vi "LIN_Config.vi"(10 "Data":T2={"Communication message"={"Sender"="", "receiver"="", "message"="", "data"=variant}, "LIN_Data"={"DLL_PATH"=path "", "Channels used"=1, "Funtiontype"=0, "Rx/TX"=enum."Rx", "Read message type"=enum."Receive&send messages", "async&sync"=enum."async", "sync_sendTimeout"=0, "LIN_SendHead"={"ALINIdxchn"=0, "ALINId"=0, "ALINDLC"=0}, "LIN_Set"={"Hardware Type"=2, "Hardware Subtype"=enum."TC1016", "AHwChannel"=0, "AAppChannel"=19, "ABaudrateKbps"=19.2, "AProtocol"=2, "AldHW"=0}, "LIN_DATA"={"Data0"=0, "Data1"=0, "Data2"=0, "Data3"=0, "Data4"=0, "Data5"=0, "Data6"=0, "Data7"=0}, "LIN_Set_Array"=[], "LDF"={"LDF Path"=path "", "LDF loading channel"=0}, "Blf_Log"={"Blf_Log_PATH"=path ""}, "LIN Scheduling Table Array"=[], "REC_Channel"=0}, "LIN Data array"=[], "error in"={"status"=FALSE, "code"=0, "source"=""}, "REC_Channel"=0, "AsynCall?"=FALSE, "DataBase_array"=refnum} {"REC_Channel" items=["CHN1", "CHN2", "CHN3", "CHN4", "CHN5", "CHN6", "CHN7", "CHN8", "CHN9", "CHN10", "CHN11", "CHN12", "CHN13", "CHN14", "CHN15", "CHN16", "CHN17", "CHN18", "CHN19", "CHN20", "CHN21", "CHN22", "CHN23", "CHN24", "CHN25", "CHN26", "CHN27", "CHN28", "CHN29", "CHN30", "CHN31", "CHN32"]; "LIN_Data"."REC_Channel" items=["CHN1", "CHN2", "CHN3", "CHN4", "CHN5", "CHN6", "CHN7", "CHN8", "CHN9", "CHN10", "CHN11", "CHN12", "CHN13", "CHN14", "CHN15", "CHN16", "CHN17", "CHN18", "CHN19", "CHN20", "CHN21", "CHN22", "CHN23", "CHN24", "CHN25", "CHN26", "CHN27", "CHN28", "CHN29", "CHN30", "CHN31", "CHN32"]; "LIN_Data"."LIN Scheduling Table Array"."LIN_Transmit"."Channel" items=["CHN1", "CHN2", "CHN3", "CHN4", "CHN5", "CHN6", "CHN7", "CHN8", "CHN9", "CHN10", "CHN11", "CHN12", "CHN13", "CHN14", "CHN15", "CHN16", "CHN17", "CHN18", "CHN19", "CHN20", "CHN21", "CHN22", "CHN23", "CHN24", "CHN25", "CHN26", "CHN27", "CHN28", "CHN29", "CHN30", "CHN31", "CHN32"]; "LIN_Data"."LIN Scheduling Table Array"."LIN_Transmit"."ID" format="%.0x"; "LIN_Data"."LIN Scheduling Table Array"."LIN_Transmit"."DLC" format="%.0x"; "LIN_Data"."LIN Scheduling Table Array"."LIN_Transmit"."Set_node_funtiontype" items=["MasterNode", "SlaveNode", "MonitorNote"]; "LIN_Data"."LDF"."LDF loading channel" items=["CHN1", "CHN2", "CHN3", "CHN4", "CHN5", "CHN6", "CHN7", "CHN8", "CHN9", "CHN10", "CHN11", "CHN12", "CHN13", "CHN14", "CHN15", "CHN16", "CHN17", "CHN18", "CHN19", "CHN20", "CHN21", "CHN22", "CHN23", "CHN24", "CHN25", "CHN26", "CHN27", "CHN28", "CHN29", "CHN30", "CHN31", "CHN32"]; "LIN_Data"."LIN_Set_Array"."Set_node_funtiontype" items=["MasterNode", "SlaveNode", "MonitorNote"]; "LIN_Data"."LIN_Set_Array"."Set"."Hardware Type" items=["BUS_UNKNOWN_TYPE", "TS_TCP_DEVICE", "XL_USB_DEVICE", "TS_USB_DEVICE", "PEAK_USB_DEVICE", "KVASER_USB_DEVICE", "ZLG_USB_DEVICE", "ICS_USB_DEVICE", "TS_TC1005_DEVICE", "CANABLE_USB_DEVICE", "TS_WIRELESS_OBD", "TS_USB_DEVICE_EX", "IXXAT_USB_DEVICE", "TS_ETH_IF_DEVICE", "TS_USB_IF_DEVICE", "BUS_DEV_TYPE_COUNT"]; "LIN_Data"."LIN_Set_Array"."Set"."AHwChannel" items=["CHN1", "CHN2", "CHN3", "CHN4", "CHN5", "CHN6", "CHN7", "CHN8", "CHN9", "CHN10", "CHN11", "CHN12", "CHN13", "CHN14", "CHN15", "CHN16", "CHN17", "CHN18", "CHN19", "CHN20", "CHN21", "CHN22", "CHN23", "CHN24", "CHN25", "CHN26", "CHN27", "CHN28", "CHN29", "CHN30", "CHN31", "CHN32"]; "LIN_Data"."LIN_Set_Array"."Set"."AAppChannel" items=["CHN1", "CHN2", "CHN3", "CHN4", "CHN5", "CHN6", "CHN7", "CHN8", "CHN9", "CHN10", "CHN11", "CHN12", "CHN13", "CHN14", "CHN15", "CHN16", "CHN17", "CHN18", "CHN19", "CHN20", "CHN21", "CHN22", "CHN23", "CHN24", "CHN25", "CHN26", "CHN27", "CHN28", "CHN29", "CHN30", "CHN31", "CHN32"]; "LIN_Data"."LIN_Set_Array"."Set"."AProtocol" items=["Lin_Protocol_13", "Lin_Protocol_20", "Lin_Protocol_21", "Lin_Protocol_J2602"]; "LIN_Data"."Funtiontype" items=["MasterNode", "SlaveNode", "MonitorNote"]; "LIN_Data"."LIN_SendHead"."ALINDLC" format="%.0x"; "LIN_Data"."LIN_SendHead"."ALINId" format="%.0x"; "LIN_Data"."LIN_SendHead"."ALINIdxchn" items=["CHN1", "CHN2", "CHN3", "CHN4", "CHN5", "CHN6", "CHN7", "CHN8", "CHN9", "CHN10", "CHN11", "CHN12", "CHN13", "CHN14", "CHN15", "CHN16", "CHN17", "CHN18", "CHN19", "CHN20", "CHN21", "CHN22", "CHN23", "CHN24", "CHN25", "CHN26", "CHN27", "CHN28", "CHN29", "CHN30", "CHN31", "CHN32"]; "LIN_Data"."LIN_Set"."Hardware Type" items=["BUS_UNKNOWN_TYPE", "TS_TCP_DEVICE", "XL_USB_DEVICE", "TS_USB_DEVICE", "PEAK_USB_DEVICE", "KVASER_USB_DEVICE", "ZLG_USB_DEVICE", "ICS_USB_DEVICE", "TS_TC1005_DEVICE", "CANABLE_USB_DEVICE", "TS_WIRELESS_OBD", "TS_USB_DEVICE_EX", "IXXAT_USB_DEVICE", "TS_ETH_IF_DEVICE", "TS_USB_IF_DEVICE", "BUS_DEV_TYPE_COUNT"]; "LIN_Data"."LIN_Set"."AHwChannel" items=["CHN1", "CHN2", "CHN3", "CHN4", "CHN5", "CHN6", "CHN7", "CHN8", "CHN9", "CHN10", "CHN11", "CHN12", "CHN13", "CHN14", "CHN15", "CHN16", "CHN17", "CHN18", "CHN19", "CHN20", "CHN21", "CHN22", "CHN23", "CHN24", "CHN25", "CHN26", "CHN27", "CHN28", "CHN29", "CHN30", "CHN31", "CHN32"]; "LIN_Data"."LIN_Set"."AAppChannel" items=["CHN1", "CHN2", "CHN3", "CHN4", "CHN5", "CHN6", "CHN7", "CHN8", "CHN9", "CHN10", "CHN11", "CHN12", "CHN13", "CHN14", "CHN15", "CHN16", "CHN17", "CHN18", "CHN19", "CHN20", "CHN21", "CHN22", "CHN23", "CHN24", "CHN25", "CHN26", "CHN27", "CHN28", "CHN29", "CHN30", "CHN31", "CHN32"]; "LIN_Data"."LIN_Set"."AProtocol" items=["Lin_Protocol_13", "Lin_Protocol_20", "Lin_Protocol_21", "Lin_Protocol_J2602"]; "LIN_Data"."Channels used" items=["1 Channel"=1, "2 Channels"=2, "3 Channels"=3, "4 Channels"=4, "5 Channels"=5]}, 11 "Queue Name":string="LIN_Config_0") -> ()   [LabVIEW 2014]
uses:
  Typedef/TSLIN_SetData.ctl
  <vilib>/Utility/miscctls.llb/LVPointTypeDef.ctl
  Utilities/Typedef/Hardware_Subtype.ctl
  <vilib>/Utility/miscctls.llb/LVPositionTypeDef.ctl
  Typedef/TLibLIN.ctl
  Typedef/TSLIN_SendHead.ctl
  Typedef/TSLIN_Config.ctl
  Typedef/TSLIN_Data.ctl
  Typedef/TSLIN_Transmit.ctl
  Typedef/TSLIN_LIN Schedule_Table.ctl
  Typedef/TSLIN_LIN_Set.ctl
  All_Control/Typedef/Hardware Type.ctl
  All_Control/Typedef/Blf_Log.ctl
  DataBase/Typedef/DataBase_array_index.ctl
  DataBase/Typedef/CAN/TCANSignal.ctl
  DataBase/Typedef/LIN/TLINSignal.ctl
  DataBase/Typedef/FlexRay/TFlexRaySignal.ctl
  DataBase/Typedef/TDBSignalProperties.ctl
  DataBase/Typedef/TDBFrameProperties.ctl
  DataBase/Typedef/TDBECUProperties.ctl
  DataBase/Typedef/TDBProperties.ctl
  DataBase/Typedef/DataBase_array.ctl
panel:
  in  "选项卡控件":T1(tab)
  in  "Channels used":u16(ring)=1 items=["1 Channel"=1, "2 Channels"=2, "3 Channels"=3, "4 Channels"=4, "5 Channels"=5, "6 Channels"=6, "7 Channels"=7, "8 Channels"=8, "9 Channels"=9, "10 Channels"=10, "11 Channels"=11, "12 Channels"=12, "13 Channels"=13, "14 Channels"=14, "15 Channels"=15]
  out "Connect ?":bool
  in  "Disconnect":bool
  in  "Connect":bool
  in  "Config":bool
  in  "DLL_PATH":path=path "C:/Program Files (x86)/TOSUN/TSMaster/bin/TSMaster.dll"
  in  "STOP":bool
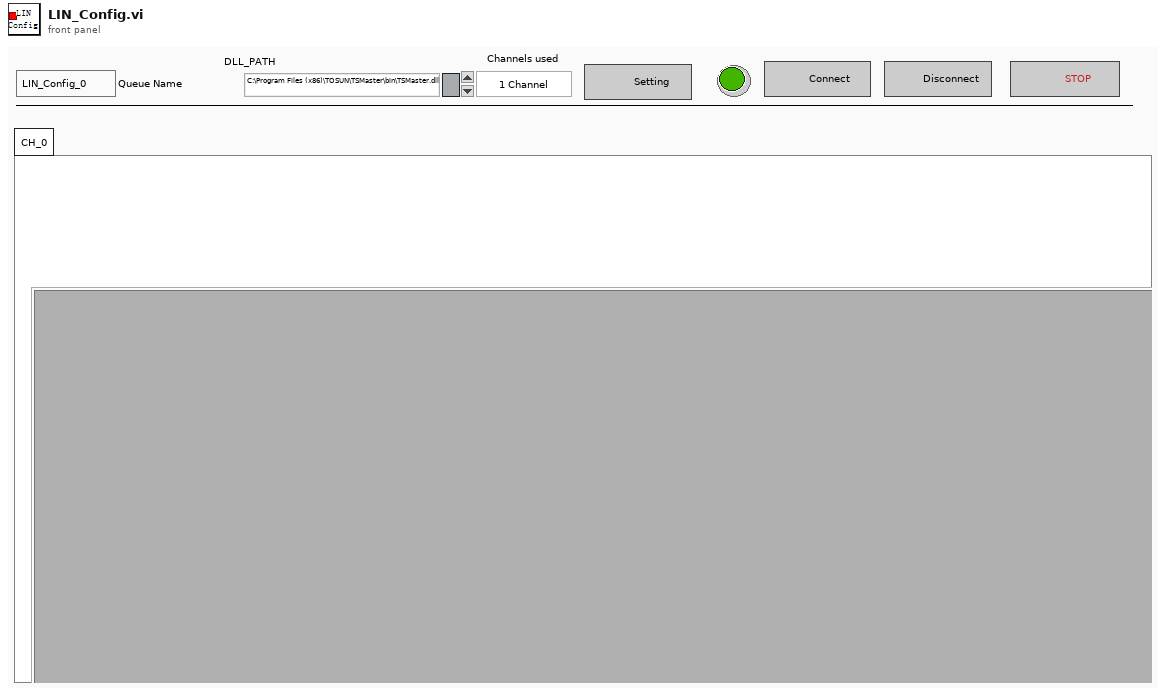
[diagram p1: front panel]
types:
  T1 = enum32{"CH_0", "CH_1", "CH_2", "CH_3", "CH_4", "CH_5", "CH_6", "CH_7", "CH_8", "CH_9", "CH_10", "CH_11", "CH_12", "CH_13", "CH_14", "CH_15"}
  T2 = typedef "TSLIN_Data.ctl" = cluster{"Communication message":cluster{"Sender":string, "receiver":string, "message":string, "data":variant}, "LIN_Data":T3, "LIN Data array":T12[], "error in":errorcluster, "REC_Channel":i32, "AsynCall?":bool, "DataBase_array":T13}
  T3 = typedef "TSLIN_Config.ctl" = cluster{"DLL_PATH":path, "Channels used":u16, "Funtiontype":i32, "Rx/TX":enum16{"Rx", "Tx"}, "Read message type":enum16{"Only read received messages", "Receive&send messages"}, "async&sync":enum16{"async", "sync"}, "sync_sendTimeout":u16, "LIN_SendHead":T4, "LIN_Set":T5, "LIN_DATA":cluster{"Data0":u8, "Data1":u8, "Data2":u8, "Data3":u8, "Data4":u8, "Data5":u8, "Data6":u8, "Data7":u8}, "LIN_Set_Array":T8[], "LDF":cluster{"LDF Path":path, "LDF loading channel":i32}, "Blf_Log":T9, "LIN Scheduling Table Array":T10[], "REC_Channel":i32}
  T4 = typedef "TSLIN_SendHead.ctl" = cluster{"ALINIdxchn":u8, "ALINId":u32, "ALINDLC":u32}
  T5 = typedef "TSLIN_SetData.ctl" = cluster{"Hardware Type":T6, "Hardware Subtype":T7, "AHwChannel":i32, "AAppChannel":i32, "ABaudrateKbps":sgl, "AProtocol":i32, "AldHW":i32}
  T6 = typedef "Hardware Type.ctl" = i32
  T7 = typedef "Hardware_Subtype.ctl" = enum16{"TS_UNKNOWN_DEVICE", "TSCAN_PRO", "TSCAN_Lite1", "TC1001", "TL1001", "TC1011", "TM5011", "TC1002", "TC1014", "TSCANFD2517", "TC1026", "TC1016", "TC1012", "TC1013", "TLog1002", "TC1034", "TC1018", "GW2116", "TC2115", "MP1013", "TC1113", "TC1114", "TP1013", "TC1017", "TP1018", "TF10XX", "TL1004_FD_4_LIN_2", "TE1051", "TP1051", "TP1034", "TTS9015", "TP1026", "TTS1026", "TTS1034", "TTS1018", "TL1011", "TTS1015_LiAuto", "TTS1013_LiAuto", "TTS1016Pro", "TC1054Pro", "TC1054", "TLog1038", "TO1013", "TC1034Pro", "TC1018Pro", "TC1038Pro", "TS_DEV_END"}
  T8 = typedef "TSLIN_LIN_Set.ctl" = cluster{"Set":T5, "Set_node_funtiontype":i32}
  T9 = typedef "Blf_Log.ctl" = cluster{"Blf_Log_PATH":path}
  T10 = typedef "TSLIN_LIN Schedule_Table.ctl" = cluster{"LIN_Transmit":T11, "Delay(ms)":i32}
  T11 = typedef "TSLIN_Transmit.ctl" = cluster{"Channel":i32, "Rx/TX":enum16{"Rx", "Tx"}, "Set_node_funtiontype":i32, "DLC":u32, "ID":u32, "FDatas":cluster{"value0":u8, "value 1":u8, "value 2":u8, "value 3":u8, "value 4":u8, "value 5":u8, "value 6":u8, "value 7":u8}}
  T12 = typedef "TLibLIN.ctl" = cluster{"Ch":u8, "Code":u8, "Properties":u8, "FDLC":u8, "ID":u8, "Checksum":u8, "FStaus":u8, "FTimeUS":u64, "FDatas":cluster{"value0":u8, "value 1":u8, "value 2":u8, "value 3":u8, "value 4":u8, "value 5":u8, "value 6":u8, "value 7":u8}}
  T13 = typedef "DataBase_array_index.ctl" = refnum<vi>
  T14 = typedef "LVPositionTypeDef.ctl" = cluster{"Left":i32, "Top":i32}
  T15 = typedef "LVPointTypeDef.ctl" = cluster{"Horizontal":i16, "Vertical":i16}
  T16 = cluster{"Sender":string, "receiver":string, "message":string, "data":variant}
  T17 = enum32{"invalid app kind", "Development System", "Run Time System", "Student Edition", "Embedded LabVIEW", "Evaluation", "Custom"}
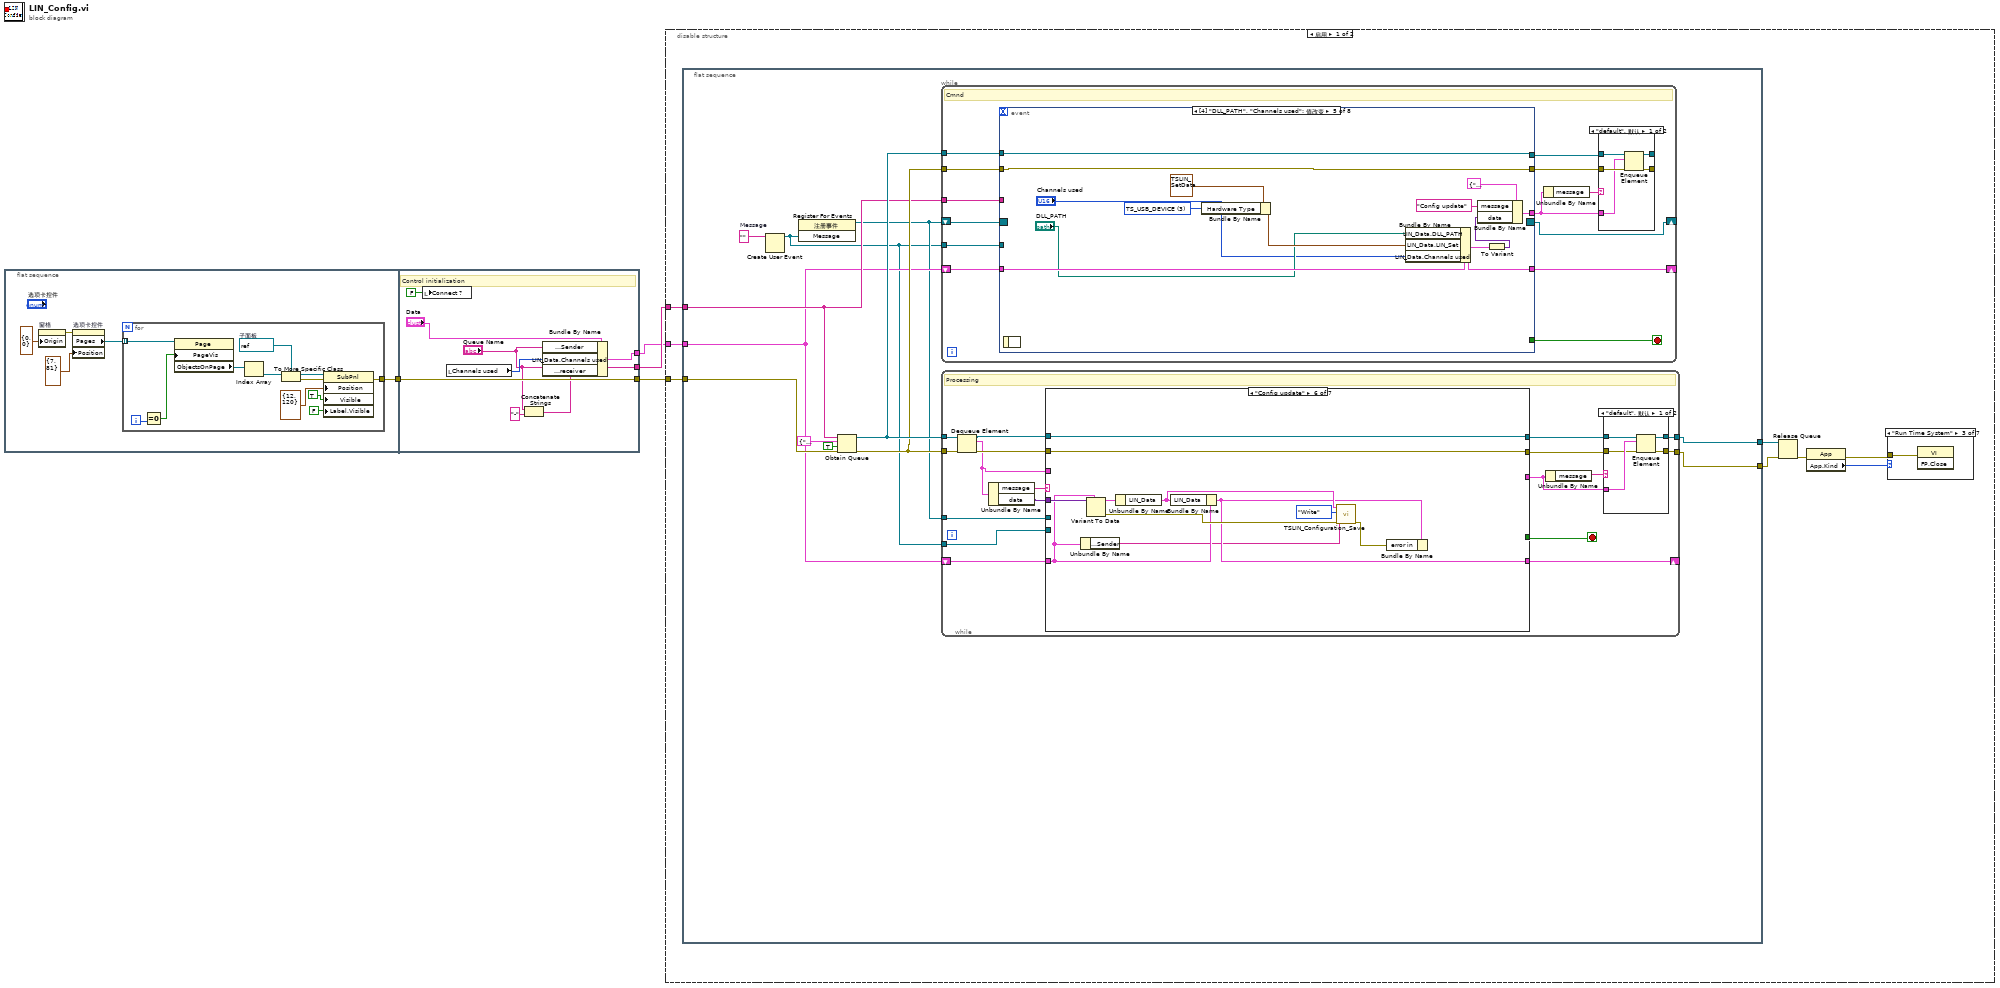
[diagram p0: block diagram]
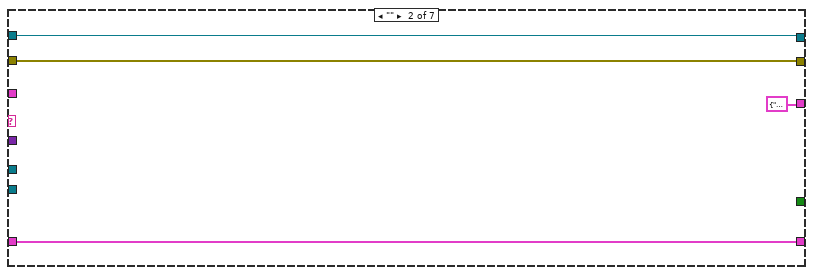
[diagram p10: hidden frame]
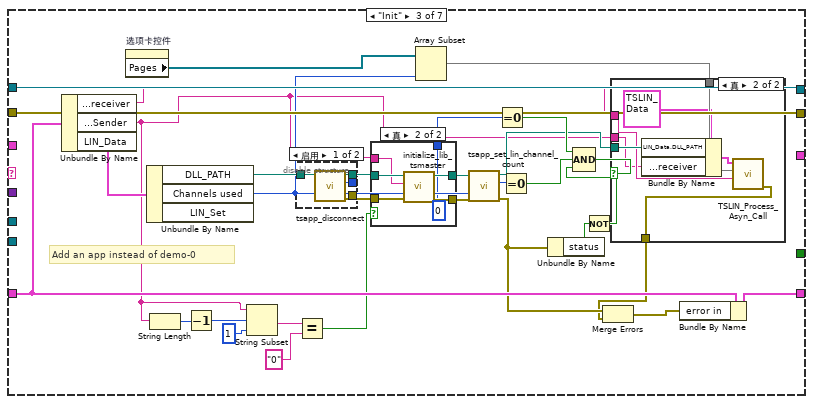
[diagram p11: hidden frame]
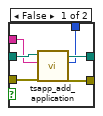
[diagram p13: hidden frame]
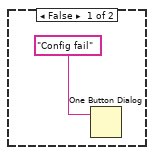
[diagram p14: hidden frame]
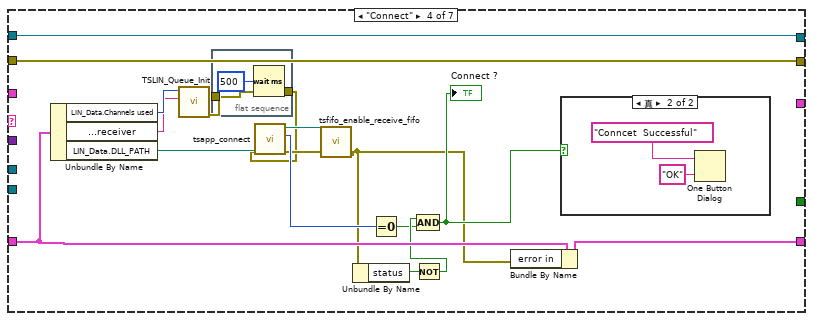
[diagram p15: hidden frame]
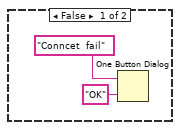
[diagram p16: hidden frame]
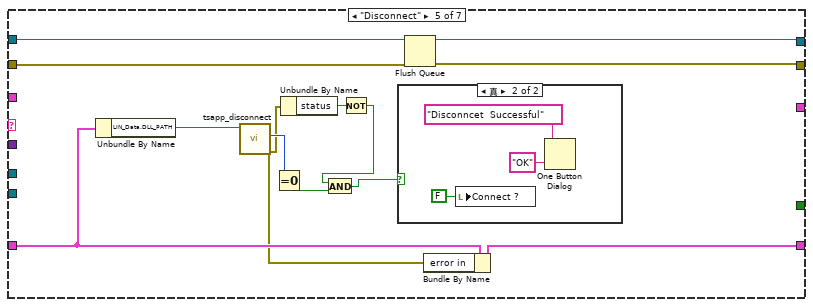
[diagram p17: hidden frame]
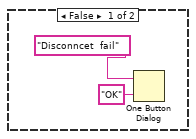
[diagram p18: hidden frame]
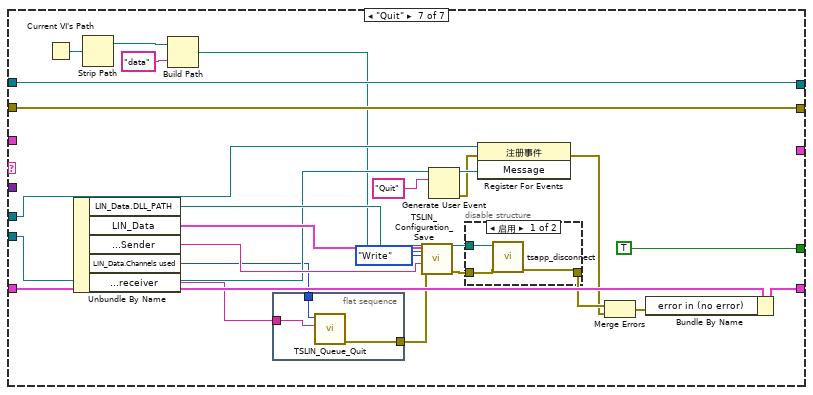
[diagram p19: hidden frame]
diagram:
  n1 = flat-sequence {
    tunnel: [w5] -> w1
    tunnel: [w26] -> w4
    tunnel: ["Queue Name"] -> w3
    tunnel: [w29] -> w2
    tunnel: w1 -> [w26]
    frame #0 {
      n2 = property on="窗格" class="Pane"("Origin"=T15 {"Horizontal"=0, "Vertical"=0} ("原点")) -> (error out=w9:errorcluster)  [unwired: 2 in, 1 out]
      n3 = property on="选项卡控件" class="TabCtl (严格)"(error in=w9, "Position"=T14 {"Left"=7, "Top"=81} ("位置")) -> ("Pages"=w8:refnum<vi>[])  [unwired: 1 in, 2 out]
      n4 = for {
        tunnel: w8 -> [w21] mode=indexing
        tunnel: [w14] -> w5
        i -> [w11]
        w19 = refnum<vi> refnum  # 子面板
        n5 = Equal To 0?(x=w11) -> (x = 0?=w10:bool)
        n6 = property class="Page"(reference=w21, "PageVis"=w10) -> ("ObjectsOnPage"=w15:refnum<vi>[])  [unwired: 1 in, 2 out]
        n7 = Index Array(array=w15) -> (element=w20:refnum<vi>)  [unwired: 1 in]
        n8 = To More Specific Class(target class=w19, reference=w20) -> (specific class reference=w18:refnum<vi>, error out=w17:errorcluster)  [unwired: 1 in]
        n9 = property class="SubPnl"(reference=w18, error in=w17, "Position"=T14 {"Left"=12, "Top"=120} ("位置"), "Visible"=TRUE ("可见"), "Label.Visible"=FALSE ("标签.可见")) -> (error out=w14:errorcluster)  [unwired: 1 out]
      }
    }
    frame #1 {
      # "Control initialization"
      n10 = local write "Connect ?"(FALSE ("Connect ?")) -> ()
      n11 = local read "Channels used"() -> (w25:u16)
      n12 = Concatenate Strings("Queue Name", "-" ("字符串")) -> (w22:string)
      n13 = Bundle By Name(cluster="Data", "Communication message.Sender"="Queue Name", "LIN_Data.Channels used"=w25, "Communication message.receiver"=w22) -> (w29:T2)
    }
  }
  n14 = disable-structure shown="启用" {
    disable-tunnel: w4 -> [w35 _]
    disable-tunnel: w3 -> [w34 _]
    disable-tunnel: w2 -> [w33 _]
    frame Enabled {
      n15 = flat-sequence {
        tunnel: w35 -> [w49]
        tunnel: w34 -> [w44]
        tunnel: w33 -> [w43]
        tunnel: [w40] -> w31
        tunnel: [w39] -> w30
        frame #0 {
          w50 = ""  # Message
          n16 = Create User Event(user event datatype=w50) -> (user event=w41:refnum<user-event>)  [unwired: 1 in, 1 out]
          n17 = register-events(w41) -> (reference out=w42:refnum<event-registration>)  [unwired: 2 in, 1 out]
          n18 = Obtain Queue(name (unnamed)=w44, element data type=T16 {"Sender"="", "receiver"="", "message"="", "data"=variant} ("Communication message"), create if not found? (T)=TRUE ("如未找到则创建？(T)"), error in (no error)=w49) -> (queue out=w48:refnum<queue>, error out=w47:errorcluster)  [unwired: 1 in, 1 out]
          n19 = while {
            tunnel: w48 -> [w235]
            tunnel: w47 -> [w233]
            tunnel: w44 -> [w229]
            shift-right: [w226] -> _
            shift-left: w43 -> [w227]
            shift-right: [w225] -> _
            shift-left: w42 -> [w228]
            tunnel: w41 -> [w224]
            stop <- w236 stop-if-true
            # "Cmnd"
            n20 = event shown="[4] \"DLL_PATH\", \"Channels used\": 值改变" {
              selector: w228 -> [_ _ _ _ _ _ _ _]
              dyn-events: [_ _ _ _ _ _ _ _] -> w225
              timeout: _ -> [_ _ _ _ _ _ _ _]
              tunnel: [_ _ _ _ _ w278 w288 TRUE ("放弃？")] -> w236
              tunnel: w235 -> [w246 w253 w257 w261 w274 w281 w287 w294]
              tunnel: [w246 w253 w257 w261 w274 w281 w287 w294] -> w234
              tunnel: [_ w251 T16 {"Sender"="", "receiver"="", "message"="Connect", "data"=variant} ("Communication message") T16 {"Sender"="", "receiver"="", "message"="Disconnect", "data"=variant} ("Communication message") w268 T16 {"Sender"="", "receiver"="", "message"="eee", "data"=variant} ("Communication message") w283 T16 {"Sender"="", "receiver"="", "message"="Quit", "data"=variant} ("Communication message")] -> w231
              tunnel: [w245 w247 w256 w260 w264 w276 w285 w292] -> w232
              tunnel: w233 -> [w245 w247 w256 w260 w264 w276 w285 w292]
              tunnel: w229 -> [_ _ _ _ _ _ _ _]
              tunnel: w227 -> [w244 w248 w255 w259 w273 w277 w286 w293]
              tunnel: [w244 w248 w255 w259 w267 w277 w286 w293] -> w226
              tunnel: w224 -> [_ _ _ _ _ _ _ _]
              event Timeout {
                n21 = event-data() -> ()  [unwired: 1 in, 3 out]
              }
              event "Config": Value Change {
                n22 = event-data() -> ()  [unwired: 1 in, 1 out]
                n23 = To Variant(anything=w248) -> (Variant=w249:variant)
                n24 = Bundle By Name(cluster=T16 {"Sender"="", "receiver"="", "message"="", "data"=variant} ("Communication message"), "message"="Init", "data"=w249) -> (w251:T16)
              }
              event "Connect": Value Change {
                n25 = event-data() -> ()  [unwired: 1 in, 1 out]
              }
              event "Disconnect": Value Change {
                n26 = event-data() -> ()  [unwired: 1 in, 1 out]
              }
              event "DLL_PATH", "Channels used": Value Change {
                w271 = 3 items=["BUS_UNKNOWN_TYPE", "TS_TCP_DEVICE", "XL_USB_DEVICE", "TS_USB_DEVICE", "PEAK_USB_DEVICE", "KVASER_USB_DEVICE", "ZLG_USB_DEVICE", "ICS_USB_DEVICE", "TS_TC1005_DEVICE"] ("硬件类型")
                n27 = event-data() -> ()  [unwired: 1 in, 1 out]
                n28 = Bundle By Name(cluster=T5 {"Hardware Type"=3, "Hardware Subtype"=enum."TC1026", "AHwChannel"=0, "AAppChannel"=0, "ABaudrateKbps"=19.2, "AProtocol"=2, "AldHW"=0} ("Set"), "Hardware Type"=w271) -> (w270:T5)
                n29 = Bundle By Name(cluster=w273, "LIN_Data.DLL_PATH"="DLL_PATH", "LIN_Data.LIN_Set"=w270, "LIN_Data.Channels used"="Channels used") -> (w267:T2)
                n30 = To Variant(anything=w267) -> (Variant=w266:variant)
                n31 = Bundle By Name(cluster=T16 {"Sender"="", "receiver"="", "message"="", "data"=variant} ("Communication message"), "message"="Config update", "data"=w266) -> (w268:T16)
              }
              event User Event {
                n32 = event-data() -> ("Message"=w280:string)  [unwired: 1 in]
                n33 = Equal?(x=w280, y="Quit") -> (x = y?=w278:bool)
              }
              event Panel Close? {
                w288 = TRUE ("放弃？")
                n34 = event-data() -> ()  [unwired: 1 in, 4 out]
                n35 = Bundle By Name(cluster=T16 {"Sender"="", "receiver"="", "message"="", "data"=variant} ("Communication message"), "message"="Quit") -> (w283:T16)
                n36 = event-data("Discard?"=w288) -> ()  [unwired: 1 in, 1 out]
              }
              event "STOP": Value Change {
                n37 = event-data() -> ()  [unwired: 1 in, 1 out]
                n38 = property on="选项卡控件" class="TabCtl (严格)"() -> (error out=w289:errorcluster, "Pages"=w290:refnum<vi>[])  [unwired: 2 in, 1 out]
                n39 = for {
                  tunnel: w290 -> [w299] mode=indexing
                  tunnel: w289 -> [w296]
                  i -> [w298]
                  n40 = Equal To 0?(x=w298) -> (x = 0?=w297:bool)
                  n41 = property class="Page" props=["ControlsOnPage", "PageVis"](reference=w299, error in=w296, "PageVis"=w297) -> ()  [unwired: 3 out]
                }
              }
            }
            n42 = Unbundle By Name(w231) -> ("message"=w230:string)
            n43 = case shown="\"default\", 默认" w230 {
              tunnel: w234 -> [w241 w243]
              tunnel: w232 -> [w240 w242]
              tunnel: w231 -> [w237 _]
              tunnel: [w239 w243] -> _
              tunnel: [w238 w242] -> _
              frame "default", Default {
                n44 = Enqueue Element(queue=w241, element=w237, error in (no error)=w240) -> (queue out=w239:refnum<queue>, error out=w238:errorcluster)  [unwired: 1 in, 1 out]
              }
              frame "" {
              }
            }
          }
          n45 = while {
            tunnel: w48 -> [w68]
            tunnel: w47 -> [w67]
            tunnel: [w60] -> w40
            tunnel: [w59] -> w39
            shift-right: [w55] -> _
            shift-left: w43 -> [w56]
            tunnel: w42 -> [w54]
            tunnel: w41 -> [w51]
            stop <- w58 stop-if-true
            # "Processing"
            n46 = Dequeue Element(queue=w68, error in (no error)=w67) -> (queue out=w65:refnum<queue>, element=w53:T16, error out=w64:errorcluster)  [unwired: 1 in, 1 out]
            n47 = Unbundle By Name(w53) -> ("message"=w66:string, "data"=w61:variant)
            n48 = case shown="\"Config update\"" w66 {
              tunnel: [w78 w82 w114 w156 w167 w189 w215] -> w63
              tunnel: w65 -> [w78 w82 w114 w156 w175 w189 w215]
              tunnel: w64 -> [w77 w81 w111 w155 w166 w188 w214]
              tunnel: [w77 w81 w111 w155 w165 w188 w214] -> w62
              tunnel: w61 -> [_ _ _ _ _ w191 _]
              tunnel: [_ _ _ _ _ _ TRUE] -> w58
              tunnel: [w76 w80 w110 w152 w172 w183 w210] -> w55
              tunnel: w56 -> [w76 w80 w112 w154 w174 w182 w212]
              tunnel: w54 -> [_ _ _ _ _ _ w203]
              tunnel: [_ T16 {"Sender"="", "receiver"="", "message"="", "data"=variant} ("Communication message") _ _ _ _ _] -> w52
              tunnel: w53 -> [_ _ _ _ _ _ _]
              tunnel: w51 -> [_ _ _ _ _ _ w202]
              frame "eee", Default {
              }
              frame "" {
              }
              frame "Init" {
                # "Add an app instead of demo-0"
                n49 = Unbundle By Name(w112) -> ("Communication message.receiver"=w92:string, "Communication message.Sender"=w86:string, "LIN_Data"=w113:T3)
                n50 = property on="选项卡控件" class="TabCtl (严格)"() -> ("Pages"=w96:refnum<vi>[])  [unwired: 2 in, 2 out]
                n51 = Unbundle By Name(w113) -> ("DLL_PATH"=w99:path, "Channels used"=w95:u16)  [unwired: 1 out]
                n52 = String Length(string=w86) -> (length=w88:i32)
                n53 = Decrement(x=w88) -> (x-1=w87:i32)
                n54 = String Subset(string=w86, offset (0)=w87, length (rest)=1 ("长度（剩余）")) -> (substring=w85:string)
                n55 = disable-structure shown="启用" {
                  disable-tunnel: w99 -> [w118 w119]
                  disable-tunnel: [w117 w119] -> w98
                  disable-tunnel: [w116 _] -> w97
                  disable-tunnel: [w115 _] -> _
                  frame Enabled {
                    n56 = call "tsapp_disconnect.vi"("Path"=w118) -> ("error output"=w116:errorcluster, "retuen"=w115:i32, "Path output"=w117:path)  [unwired: 8 in]
                  }
                  frame Disabled {
                  }
                }
                n57 = Equal?(x=w85, y="0" ("正则表达式")) -> (x = y?=w83:bool)
                n58 = case shown="真" w83 {
                  tunnel: w98 -> [w125 w131]
                  tunnel: w86 -> [w122 w130]
                  tunnel: [w123 w129] -> w100
                  tunnel: [w124 w128] -> w101
                  tunnel: [w121 0 ("return")] -> w103
                  tunnel: w97 -> [w120 w126]
                  frame False {
                    n59 = call "tsapp_add_application.vi"("error in (no error)"=w120, "AAppName"=w122, "路径输入"=w125) -> ("error out"=w123:errorcluster, "retuen"=w121:i32, "路径输出"=w124:path)  [unwired: 6 in]
                  }
                  frame True {
                    n60 = call "initialize_lib_tsmaster.vi"("error in (no error)"=w126, "AppName"=w130, "Path input"=w131) -> ("error output"=w129:errorcluster, "Path output"=w128:path)  [unwired: 7 in]
                  }
                }
                n61 = Array Subset(array=w96, length=w95) -> (w94:refnum<vi>[])  [unwired: 1 in]
                n62 = call "tsapp_set_lin_channel_count.vi"("error in (no error)"=w100, "Aount"=w95, "Path"=w101) -> ("error out"=w106:errorcluster, "return"=w105:i32, "Path output"=w93:path)  [unwired: 6 in]
                n63 = Equal To 0?(x=w103) -> (x = 0?=w102:bool)
                n64 = Equal To 0?(x=w105) -> (x = 0?=w104:bool)
                n65 = Unbundle By Name(w106) -> ("status"=w109:bool)
                n66 = Not(x=w109) -> (.not. x?=w108:bool)
                n67 = Compound Arithmetic op=AND(w102, w104, w108) -> (w107:bool)
                n68 = case shown="真" w107 {
                  tunnel: w94 -> [_ w139]
                  tunnel: w93 -> [_ w136]
                  tunnel: w92 -> [_ w135]
                  tunnel: [_ w134] -> w90
                  tunnel: w86 -> [_ w133]
                  frame False {
                    n69 = One Button Dialog(message="Config fail" ("消息")) -> ()  [unwired: 1 in, 1 out]
                  }
                  frame True {
                    n70 = Bundle By Name(cluster=T2 {"Communication message"={"Sender"="", "receiver"="", "message"="", "data"=variant}, "LIN_Data"={"DLL_PATH"=path "", "Channels used"=1, "Funtiontype"=0, "Rx/TX"=enum."Rx", "Read message type"=enum."Receive&send messages", "async&sync"=enum."async", "sync_sendTimeout"=0, "LIN_SendHead"={"ALINIdxchn"=0, "ALINId"=0, "ALINDLC"=0}, "LIN_Set"={"Hardware Type"=2, "Hardware Subtype"=enum."TC1016", "AHwChannel"=0, "AAppChannel"=19, "ABaudrateKbps"=19.2, "AProtocol"=2, "AldHW"=0}, "LIN_DATA"={"Data0"=0, "Data1"=0, "Data2"=0, "Data3"=0, "Data4"=0, "Data5"=0, "Data6"=0, "Data7"=0}, "LIN_Set_Array"=[], "LDF"={"LDF Path"=path "", "LDF loading channel"=0}, "Blf_Log"={"Blf_Log_PATH"=path ""}, "LIN Scheduling Table Array"=[], "REC_Channel"=0}, "LIN Data array"=[], "error in"={"status"=FALSE, "code"=0, "source"=""}, "REC_Channel"=0, "AsynCall?"=FALSE, "DataBase_array"=refnum} ("Data"), "LIN_Data.DLL_PATH"=w136, "Communication message.receiver"=w133) -> (w137:T2)
                    n71 = call "TSLIN_Process_Asyn_Call.vi"("Queue Name"=w135, "Ref_Arry"=w139, "Data"=w137) -> ("error out"=w134:errorcluster)  [unwired: 8 in]
                  }
                }
                n72 = Merge Errors(w106, w90) -> (w91:errorcluster)
                n73 = Bundle By Name(cluster=w112, "error in"=w91) -> (w110:T2)
              }
              frame "Connect" {
                n74 = Unbundle By Name(w154) -> ("LIN_Data.Channels used"=w143:u16, "Communication message.receiver"=w142:string, "LIN_Data.DLL_PATH"=w153:path)
                n75 = call "TSLIN_Queue_Init.vi"("receiver"=w142, "Channels used"=w143) -> ("error out"=w141:errorcluster)  [unwired: 9 in]
                n76 = flat-sequence {
                  tunnel: w141 -> [w158]
                  tunnel: [w158] -> w140
                  frame #0 {
                    n77 = Wait (ms)(milliseconds to wait=u32 500 ("等待时间（毫秒）")) -> ()  [unwired: 1 out]
                  }
                }
                n78 = call "tsapp_connect.vi"("error in (no error)"=w140, "Path"=w153) -> ("error out"=w144:errorcluster, "retuen"=w151:i32, "Path output"=w145:path)  [unwired: 7 in]
                n79 = call "tsfifo_enable_receive_fifo.vi"("error in (no error)"=w144, "Path"=w145) -> ("error out"=w147:errorcluster)  [unwired: 8 in, 1 out]
                n80 = Unbundle By Name(w147) -> ("status"=w149:bool)
                n81 = Equal To 0?(x=w151) -> (x = 0?=w146:bool)
                n82 = Not(x=w149) -> (.not. x?=w148:bool)
                n83 = Compound Arithmetic op=AND(w148, w146) -> (w150:bool)
                "Connect ?" <- w150
                n84 = Bundle By Name(cluster=w154, "error in"=w147) -> (w152:T2)
                n85 = case shown="真" w150 {
                  frame False {
                    n86 = One Button Dialog(message="Conncet  fail" ("消息"), button name ("OK")="OK" ("按钮名称（“确定”）")) -> ()  [unwired: 1 out]
                  }
                  frame True {
                    n87 = One Button Dialog(message="Conncet  Successful" ("消息"), button name ("OK")="OK" ("按钮名称（“确定”）")) -> ()  [unwired: 1 out]
                  }
                }
              }
              frame "Disconnect" {
                n88 = Unbundle By Name(w174) -> ("LIN_Data.DLL_PATH"=w173:path)
                n89 = call "tsapp_disconnect.vi"("Path"=w173) -> ("error output"=w163:errorcluster, "retuen"=w171:i32)  [unwired: 8 in, 1 out]
                n90 = Equal To 0?(x=w171) -> (x = 0?=w164:bool)
                n91 = Unbundle By Name(w163) -> ("status"=w169:bool)
                n92 = Not(x=w169) -> (.not. x?=w168:bool)
                n93 = And(x=w168, y=w164) -> (x .and. y?=w170:bool)
                n94 = case shown="真" w170 {
                  frame False {
                    n95 = One Button Dialog(message="Disconncet  fail" ("消息"), button name ("OK")="OK" ("按钮名称（“确定”）")) -> ()  [unwired: 1 out]
                  }
                  frame True {
                    n96 = local write "Connect ?"(FALSE ("Connect ?")) -> ()
                    n97 = One Button Dialog(message="Disconncet  Successful" ("消息"), button name ("OK")="OK" ("按钮名称（“确定”）")) -> ()  [unwired: 1 out]
                  }
                }
                n98 = Flush Queue(queue=w175, error in (no error)=w166) -> (queue out=w167:refnum<queue>, error out=w165:errorcluster)  [unwired: 1 out]
                n99 = Bundle By Name(cluster=w174, "error in"=w163) -> (w172:T2)
              }
              frame "Config update" {
                n100 = Unbundle By Name(w182) -> ("Communication message.Sender"=w181:string)
                n101 = Variant To Data(type=w182, Variant=w191) -> (data=w190:T2, error out=w185:errorcluster)  [unwired: 1 in]
                n102 = Unbundle By Name(w190) -> ("LIN_Data"=w184:T3)
                n103 = Bundle By Name(cluster=w182, "LIN_Data"=w184) -> (w183:T2)
                n104 = call "TSLIN_Configuration_Save.vi"("error in (no error)"=w185, "Config Name"=w181, "Read/Write"=enum16{"Read", "Write"}."Write", "LIN_Data"=w184) -> ("error in (no error) 2"=w186:errorcluster)  [unwired: 5 in, 2 out]
                n105 = Bundle By Name(cluster=w183, "error in"=w186) -> ()  [unwired: 1 out]
              }
              frame "Quit" {
                n106 = Current VI's Path() -> (path=w207:path)
                n107 = Unbundle By Name(w212) -> ("LIN_Data.DLL_PATH"=w208:path, "LIN_Data"=w211:T3, "Communication message.Sender"=w206:string, "LIN_Data.Channels used"=w192:u16, "Communication message.receiver"=w193:string)
                n108 = Strip Path(path=w207) -> (stripped path=w197:path)  [unwired: 1 out]
                n109 = Build Path(base path=w197, name or relative path="data") -> (appended path=w196:path)
                n110 = flat-sequence {
                  tunnel: [w217] -> w194
                  tunnel: w193 -> [w219]
                  tunnel: w192 -> [w218]
                  frame #0 {
                    n111 = call "TSLIN_Queue_Quit.vi"("receiver"=w219, "Channels used"=w218) -> ("error out"=w217:errorcluster)  [unwired: 9 in]
                  }
                }
                n112 = call "TSLIN_Configuration_Save.vi"("path"=w196, "error in (no error)"=w194, "Config Name"=w206, "Read/Write"=enum16{"Read", "Write"}."Write", "LIN_Data"=w211) -> ("error in (no error) 2"=w209:errorcluster)  [unwired: 4 in, 2 out]
                n113 = Generate User Event(user event=w202, event data cluster="Quit" ("y")) -> (user event out=w204:refnum<user-event>, error out=w200:errorcluster)  [unwired: 2 in]
                n114 = disable-structure shown="启用" {
                  disable-tunnel: w209 -> [w222 w223]
                  disable-tunnel: w208 -> [w221 _]
                  disable-tunnel: [w220 w223] -> w199
                  frame Enabled {
                    n115 = call "tsapp_disconnect.vi"("error in (no error)"=w222, "Path"=w221) -> ("error output"=w220:errorcluster)  [unwired: 7 in, 2 out]
                  }
                  frame Disabled {
                  }
                }
                n116 = register-events(reference=w203, error in=w200, w204) -> (error out=w198:errorcluster)  [unwired: 1 out]
                n117 = Merge Errors(w199, w198) -> (w201:errorcluster)
                n118 = Bundle By Name(cluster=w212, "error in (no error)"=w201) -> (w210:T2)
              }
            }
            n119 = Unbundle By Name(w52) -> ("message"=w57:string)
            n120 = case shown="\"default\", 默认" w57 {
              tunnel: w63 -> [w73 w75]
              tunnel: w62 -> [w69 w74]
              tunnel: [w72 w75] -> w60
              tunnel: [w71 w74] -> w59
              tunnel: w52 -> [w70 _]
              frame "default", Default {
                n121 = Enqueue Element(queue=w73, element=w70, error in (no error)=w69) -> (queue out=w72:refnum<queue>, error out=w71:errorcluster)  [unwired: 1 in, 1 out]
              }
              frame "" {
              }
            }
          }
        }
      }
      n122 = Release Queue(queue=w31, error in (no error)=w30) -> (error out=w32:errorcluster)  [unwired: 1 in, 2 out]
      n123 = property class="App"(error in=w32) -> (error out=w37:errorcluster, "App.Kind"=w36:T17)  [unwired: 1 in, 1 out]
      n124 = case shown="\"Run Time System\"" w36 {
        tunnel: w37 -> [_ _ w38 _ _ _ _]
        frame "invalid app kind", Default {
        }
        frame "Development System" {
        }
        frame "Run Time System" {
          n125 = invoke class="VI" method="FP.Close"(error in=w38) -> ()  [unwired: 2 in, 3 out]
        }
        frame "Student Edition" {
        }
        frame "Embedded LabVIEW" {
        }
        frame "Evaluation" {
        }
        frame "Custom" {
        }
      }
    }
    frame Disabled {
    }
  }
